vi "Setup SMU_PD and Measure Resistance Only 20220831.vi"(4 "PD_v":dbl=41.0 format="%#_13g", 5 "SMU_PD":string[](array[string])=["VDD"], 6 "Published_ID":string="_Free", 7 "Settings":T2 {"Sense" items=["Local"=1008, "Remote"=1009]}, 8 "error in (no error)":errorcluster, 9 "current level":dbl=0.01 format="%_6p", 10 "Pins":string[](array[string]), 11 "Semiconductor Module Context":T3) -> (0 "error out":errorcluster, 3 "Semiconductor Module Context Out":T3)   [LabVIEW 2013]
uses:
  <vilib>/NI_TestStand_SemiconductorModule/NI_TestStand_Semiconductor_Module.lvlibp/PinMap/General/SemiconductorModuleContext.ctl
  <instrlib>/niDCPower/nidcpower.llb/niDCPower Sense.ctl
  <instrlib>/niDCPower/nidcpower.llb/niDCPower Wait For Event - Event.ctl
  <vilib>/NI_TestStand_SemiconductorModule/NI_TestStand_Semiconductor_Module.lvlibp/PinMap/DC Power/PinToNIDCPowerSessions.vi
  <vilib>/NI_TestStand_SemiconductorModule/NI_TestStand_Semiconductor_Module.lvlibp/PinMap/General/Publish/PublishDataDoubleFunctionalTest.vi
  <vilib>/NI_TestStand_SemiconductorModule/NI_TestStand_Semiconductor_Module.lvlibp
panel:
  out "R Array":dbl[](array[numeric])
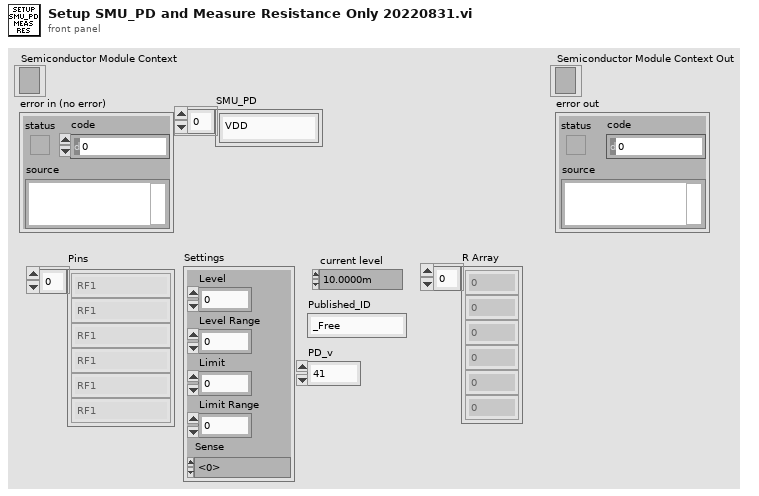
[diagram p1: front panel]
types:
  T1 = typedef "niDCPower Sense.ctl" = i32
  T2 = cluster{"Level":dbl, "Level Range":dbl, "Limit":dbl, "Limit Range":dbl, "Sense":T1}
  T3 = typedef "NI_TestStand_Semiconductor_Module.lvlibp/SemiconductorModuleContext.ctl" = refnum<k7>
  T4 = typedef "niDCPower Wait For Event - Event.ctl" = i32
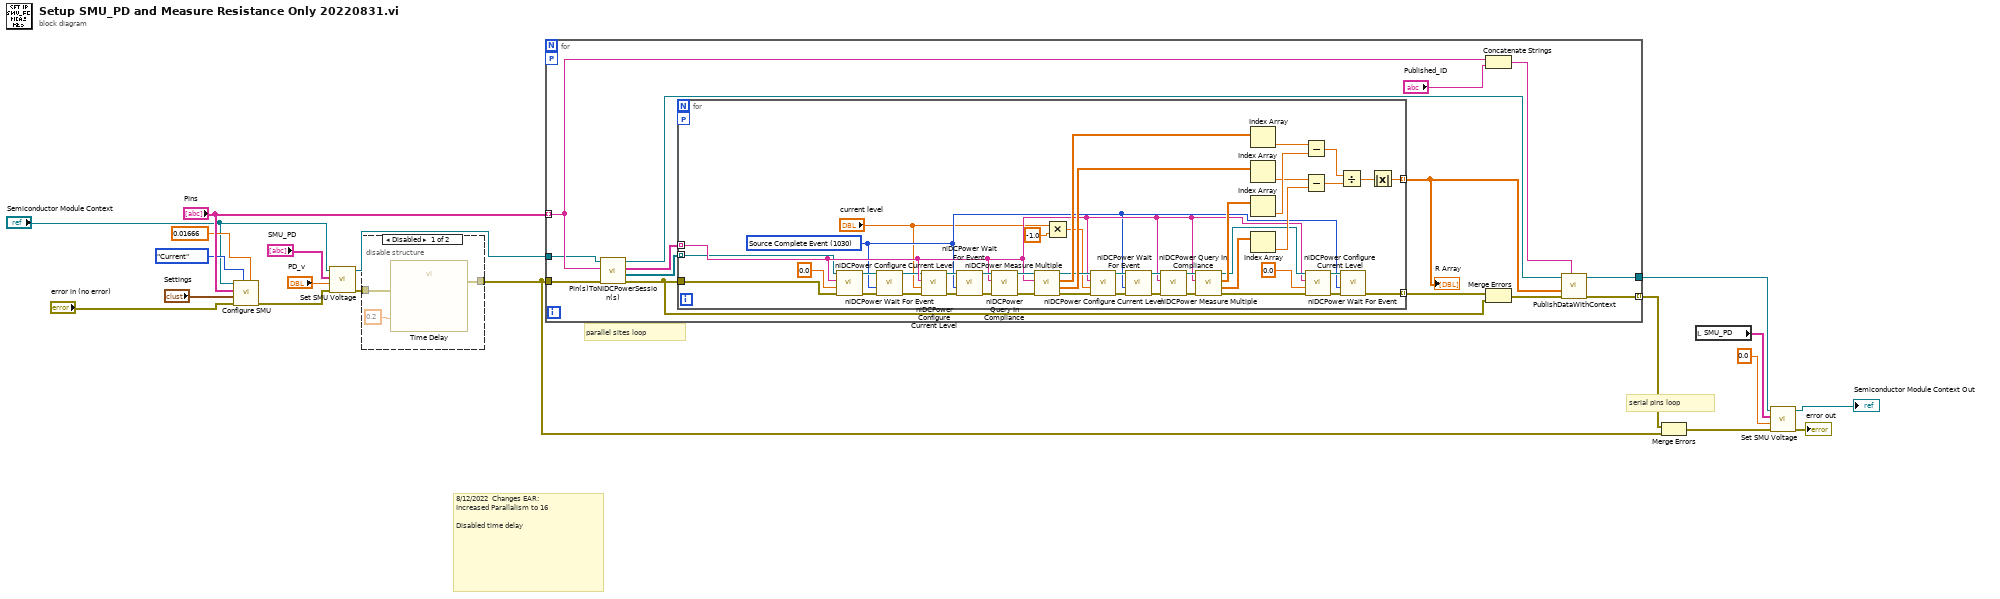
[diagram p0: block diagram]
diagram:
  # "8/12/2022  Changes EAR:\nIncreased Parallalism to 16\n\nDisabled time delay"
  # "parallel sites loop"
  # "serial pins loop"
  n1 = call "Configure SMU.vi"("aperture time"=0.01666, "Source Mode"=enum16{"Voltage", "Current"}."Current", "error in (no error)"="error in (no error)", "Settings"="Settings", "Pins"="Pins", "Semiconductor Module Context"="Semiconductor Module Context") -> ("error out"=w7:errorcluster)  [unwired: 5 in]
  n2 = call "Set SMU Voltage.vi"("error in (no error)"=w7, "VDD voltage level"="PD_v", "Pins"="SMU_PD", "Semiconductor Module Context"="Semiconductor Module Context") -> ("error out"=w8:errorcluster, "Semiconductor Module Context Out"=w1:T3)  [unwired: 5 in, 1 out]
  n3 = disable-structure shown="Disabled" {
    disable-tunnel: [w21 w23] -> w14
    disable-tunnel: w8 -> [w20 w23]
    frame Disabled {
      n4 = call "Time Delay"("error in (no error)"=w20, "Delay Time (s)"=0.2) -> ("error out"=w21:errorcluster)  [unwired: 9 in]
    }
    frame Enabled {
    }
  }
  n5 = for {
    tunnel: [w31] -> w10
    tunnel: "Pins" -> [w28] mode=indexing
    tunnel: w14 -> [w37]
    tunnel: [w29] -> w19 mode=indexing
    tunnel: w1 -> [w24]
    workers-P: _ -> [_]
    n6 = call-poly <vilib>:"Pin(s)ToNIDCPowerSession(s).vi"("error in (no error)"=w37, "Pin"=w28, "Semiconductor Module Context"=w24) -> ("error out"=w33:errorcluster, "Instrument Sessions"=w35:refnum<k15>[], "Channel Lists"=w36:string[], "Semiconductor Module Context Out"=w32:T3)  [unwired: 4 in, 1 out]
    n7 = for {
      tunnel: w36 -> [w47] mode=indexing
      tunnel: w35 -> [w46] mode=indexing
      workers-P: _ -> [_]
      tunnel: w33 -> [w49]
      tunnel: [w80] -> w34 mode=indexing
      tunnel: [w69] -> w25 mode=indexing
      w42 = T4 1030 items=["Source Complete Event"=1030, "Measure Complete Event"=1031, "Sequence Iteration Complete Event"=1032, "Sequence Engine Done Event"=1033, "Pulse Complete Event"=1051, "Ready For Pulse Trigger Event"=1052] ("event")
      n8 = call <instrlib>:"niDCPower Configure Current Level.vi"("error in (no error)"=w49, "current level"=0.0, "channel name"=w47, "instrument handle"=w46) -> ("error out"=w50:errorcluster, "instrument handle out"=w45:refnum<k15>)  [unwired: 6 in]
      n9 = call <instrlib>:"niDCPower Wait For Event.vi"("error in (no error)"=w50, "event"=w42, "instrument handle"=w45) -> ("error out"=w48:errorcluster, "instrument handle out"=w44:refnum<k15>)  [unwired: 7 in]
      n10 = call <instrlib>:"niDCPower Configure Current Level.vi"("error in (no error)"=w48, "current level"="current level", "channel name"=w47, "instrument handle"=w44) -> ("error out"=w74:errorcluster, "instrument handle out"=w73:refnum<k15>)  [unwired: 6 in]
      n11 = call <instrlib>:"niDCPower Wait For Event.vi"("error in (no error)"=w74, "event"=w42, "instrument handle"=w73) -> ("error out"=w39:errorcluster, "instrument handle out"=w79:refnum<k15>)  [unwired: 7 in]
      n12 = call <instrlib>:"niDCPower Query In Compliance.vi"("error in (no error)"=w39, "channel name"=w47, "instrument handle"=w79) -> ("error out"=w75:errorcluster, "instrument handle out"=w76:refnum<k15>)  [unwired: 6 in, 1 out]
      n13 = call <instrlib>:"niDCPower Measure Multiple.vi"("error in (no error)"=w75, "channel name"=w47, "instrument handle"=w76) -> ("error out"=w54:errorcluster, "current measurements"=w70:dbl[], "voltage measurements"=w71:dbl[], "instrument handle out"=w52:refnum<k15>)  [unwired: 5 in]
      n14 = Multiply(x="current level", y=-1.0) -> (x*y=w41:dbl)
      n15 = call <instrlib>:"niDCPower Configure Current Level.vi"("error in (no error)"=w54, "current level"=w41, "channel name"=w47, "instrument handle"=w52) -> ("error out"=w64:errorcluster, "instrument handle out"=w63:refnum<k15>)  [unwired: 6 in]
      n16 = call <instrlib>:"niDCPower Wait For Event.vi"("error in (no error)"=w64, "event"=w42, "instrument handle"=w63) -> ("error out"=w38:errorcluster, "instrument handle out"=w67:refnum<k15>)  [unwired: 7 in]
      n17 = call <instrlib>:"niDCPower Query In Compliance.vi"("error in (no error)"=w38, "channel name"=w47, "instrument handle"=w67) -> ("error out"=w65:errorcluster, "instrument handle out"=w66:refnum<k15>)  [unwired: 6 in, 1 out]
      n18 = call <instrlib>:"niDCPower Measure Multiple.vi"("error in (no error)"=w65, "channel name"=w47, "instrument handle"=w66) -> ("error out"=w53:errorcluster, "current measurements"=w61:dbl[], "voltage measurements"=w62:dbl[], "instrument handle out"=w51:refnum<k15>)  [unwired: 5 in]
      n19 = Index Array(array=w71) -> (element=w58:dbl)  [unwired: 1 in]
      n20 = Index Array(array=w70) -> (element=w57:dbl)  [unwired: 1 in]
      n21 = Index Array(array=w62) -> (element=w60:dbl)  [unwired: 1 in]
      n22 = Index Array(array=w61) -> (element=w59:dbl)  [unwired: 1 in]
      n23 = Subtract(x=w58, y=w60) -> (x-y=w56:dbl)
      n24 = Subtract(x=w57, y=w59) -> (x-y=w55:dbl)
      n25 = call <instrlib>:"niDCPower Configure Current Level.vi"("error in (no error)"=w53, "current level"=0.0, "channel name"=w47, "instrument handle"=w51) -> ("error out"=w81:errorcluster, "instrument handle out"=w78:refnum<k15>)  [unwired: 6 in]
      n26 = Divide(x=w56, y=w55) -> (x/y=w72:dbl)
      n27 = call <instrlib>:"niDCPower Wait For Event.vi"("error in (no error)"=w81, "event"=w42, "instrument handle"=w78) -> ("error out"=w80:errorcluster)  [unwired: 7 in, 1 out]
      n28 = Absolute Value(x=w72) -> (abs(x)=w69:dbl)
    }
    "R Array" <- w25
    n29 = Concatenate Strings(w28, "Published_ID") -> (w26:string)
    n30 = Merge Errors(w34, w33) -> (w30:errorcluster)
    n31 = call-poly <vilib>:"PublishDataWithContext.vi"("Published Data Id"=w26, "error in (no error)"=w30, "Data In"=w25, "Semiconductor Module Context"=w32) -> ("error out"=w29:errorcluster, "Semiconductor Module Context Out"=w31:T3)  [unwired: 6 in]
  }
  n32 = Merge Errors(w19, w14) -> (w11:errorcluster)
  n33 = local read "SMU_PD"() -> (w3:string[])
  n34 = call "Set SMU Voltage.vi"("error in (no error)"=w11, "VDD voltage level"=0.0, "Pins"=w3, "Semiconductor Module Context"=w10) -> ("error out"=→"error out":errorcluster, "Semiconductor Module Context Out"=→"Semiconductor Module Context Out":T3)  [unwired: 5 in, 1 out]
